vi "Working with Objects.vi"() -> ()   [LabVIEW 2015]
uses:
  <vilib>/NI/JSON Support for LabVIEW/JSON Data Classes/JSON Helper/JSON Helper.lvclass
  <vilib>/NI/JSON Support for LabVIEW/JSON Data Classes/JSON Object/JSON Object.lvclass
  <vilib>/NI/JSON Support for LabVIEW/JSON Data Classes/JSON Object/Insert Key Value Pair (Single String).vi
  <vilib>/NI/JSON Support for LabVIEW/JSON Data Classes/JSON Object/New JSON Object (Empty).vi
  <vilib>/NI/JSON Support for LabVIEW/JSON Data Classes/JSON Object/Set Object Parameters XNode/Set Object Parameters.xnode
panel:
  out "Keys Deleted":string
  out "found test?":bool
  out "found key1?":bool
  out "replaced":bool
  out "Zero Replaced":string
  out "Original Object":string
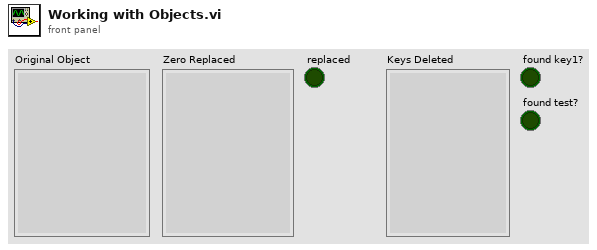
[diagram p1: front panel]
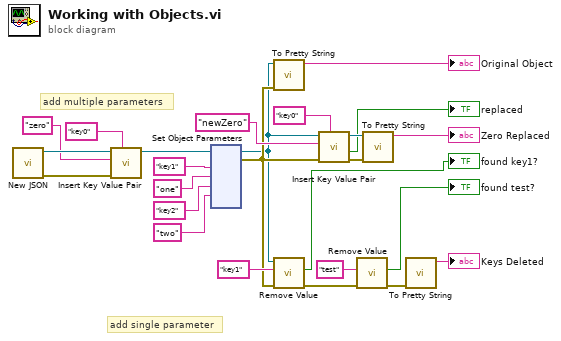
[diagram p0: block diagram]
diagram:
  # "add multiple parameters"
  # "add single parameter"
  n1 = call-poly <vilib>:"New JSON.vi"() -> ("error out"=w22:errorcluster, "JSON Object out"=w25:refnum<class "JSON Object.lvclass">)  [unwired: 10 in]
  n2 = call-poly <vilib>:"Insert Key Value Pair.vi"("key"="key0", "error in (no error)"=w22, "value"="zero" ("JSON Data in"), "JSON Object in"=w25) -> ("JSON Object out"=w7:refnum<class "JSON Object.lvclass">)  [unwired: 5 in, 2 out]
  n3 = xnode "Set Object Parameters"("key"="key1", "key"="key2", "parameter"="one" ("JSON Data in"), "parameter"="two" ("JSON Data in"), "JSON Object In"=w7) -> ("JSON Object Out"=w1:refnum<class "JSON Object.lvclass">, "error out"=w2:errorcluster)  [unwired: 1 in, 2 out]
  n4 = call-dynamic "To Pretty String.vi"("error in (no error)"=w2, "JSON Object in"=w1) -> ("Pretty Print String"=→"Original Object":string)  [unwired: 8 in, 1 out]
  n5 = call <vilib>:"Remove Value.vi"("error in (no error)"=w2, "key"="key1", "JSON Object in"=w1) -> ("error out"=w11:errorcluster, "found"=→"found key1?":bool)  [unwired: 7 in]
  n6 = call-poly <vilib>:"Insert Key Value Pair.vi"("key"="key0", "error in (no error)"=w2, "value"="newZero" ("JSON Data in"), "JSON Object in"=w1) -> ("error out"=w16:errorcluster, "replaced"=→"replaced":bool, "JSON Object out"=w17:refnum<class "JSON Object.lvclass">)  [unwired: 5 in]
  n7 = call <vilib>:"Remove Value.vi"("error in (no error)"=w11, "key"="test") -> ("error out"=w9:errorcluster, "found"=→"found test?":bool)  [unwired: 8 in]
  n8 = call-dynamic "To Pretty String.vi"("error in (no error)"=w16, "JSON Object in"=w17) -> ("Pretty Print String"=→"Zero Replaced":string)  [unwired: 8 in, 1 out]
  n9 = call-dynamic "To Pretty String.vi"("error in (no error)"=w9) -> ("Pretty Print String"=→"Keys Deleted":string)  [unwired: 9 in, 1 out]
